vi "niRFUtil RFHS Channelizer FineTuneResamplerArray CSG.vi"(0 "Resampler Ref":refnum<data-value>, 1 "Data":csg[](array[numeric]), 2 "Data Subset":T1={"Offset"=0, "Length"=-1}, 4 "fs shift (ppm)":dbl, 5 "error in (no error)":errorcluster, 6 "Reset":bool, 7 "phase shift (samples)":dbl, 8 "Requested Output Samples":i32=-1, 10 "Benchmark Task":T2, 11 "CPU Context":string) -> (14 "Resampler Ref (out)":refnum<data-value>, 15 "Resampled Data":csg[](array[numeric]), 16 "Input Samples Consumed":i32, 19 "error out":errorcluster)   [LabVIEW 2015, in "niRFUtil.lvlib"]
uses:
  niRFUtil.lvlib
  Utilities/Benchmark/niRFUtil RFHS Benchmark Task.ctl
  Utilities/niRFUtil RFHS Util Data Subset.ctl
  Includes/niRFUtil RFHS Channelizer ResamplerInfo CSG.ctl
  Includes/niRFUtil RFHS Channelizer FilterRef.ctl
  Includes/niRFUtil RFHS Channelizer ChannelizerBufferingMode.ctl
  Utilities/Data FIFO/niRFUtil RFHS FIFO Reference.ctl
  Utilities/Data FIFO/niRFUtil RFHS FIFO.ctl
  Includes/niRFUtil RFHS Channelizer ChannelizerFlags.ctl
  niRFUtil RFHS Channelizer AdjustDataSubsetSpecification.vi
  Utilities/niRFUtil RFHS Util Dll Path.vi
  niRFUtil RFHS Channelizer ProcessCPUContext.vi
  niRFUtil RFHS Channelizer ChannelizerHandleDllError.vi
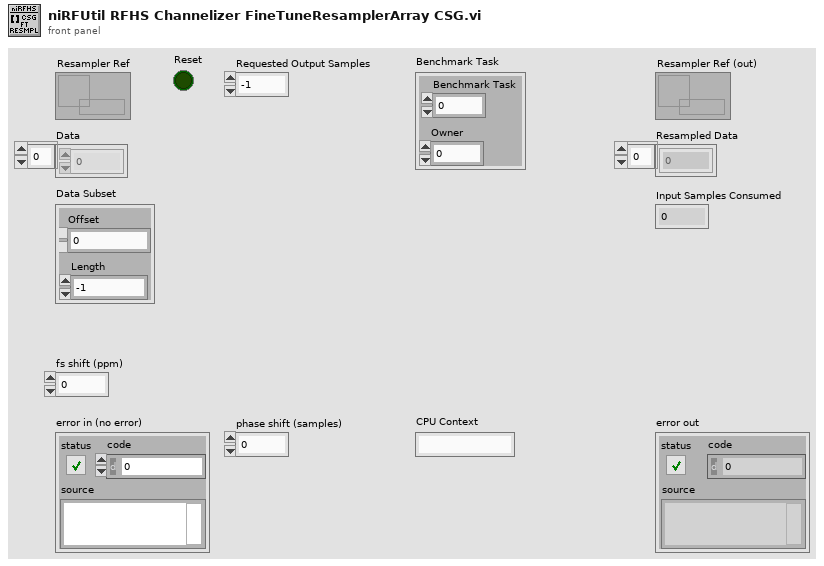
[diagram p1: front panel]
types:
  T1 = typedef "niRFUtil.lvlib/niRFUtil RFHS Util Data Subset.ctl" = cluster{"Offset":i32, "Length":i32}
  T2 = typedef "niRFUtil.lvlib/niRFUtil RFHS Benchmark Task.ctl" = cluster{"Benchmark Task":u64, "Owner":u32}
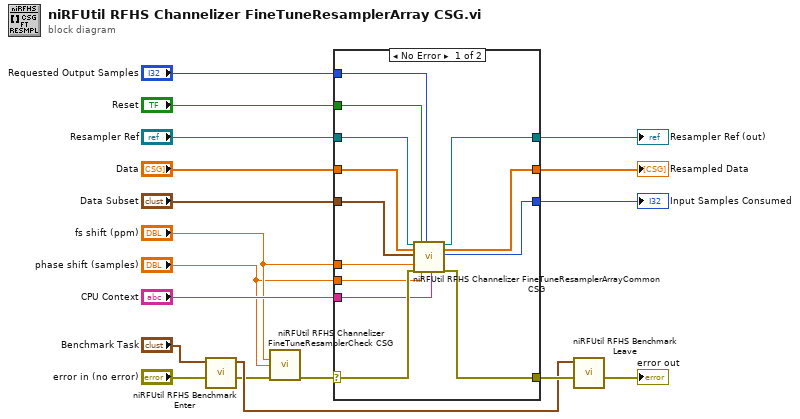
[diagram p0: block diagram]
diagram:
  n1 = call "niRFUtil RFHS Benchmark Enter.vi"("error in (no error)"="error in (no error)", "Benchmark Task (Parent)"="Benchmark Task") -> ("error out"=w4:errorcluster, "Benchmark Task (Self)"=w9:T2)  [unwired: 8 in]
  n2 = call "niRFUtil RFHS Channelizer FineTuneResamplerCheck CSG.vi"("fs shift (ppm)"="fs shift (ppm)", "phase shift (samples)"="phase shift (samples)", "error in (no error)"=w4) -> ("error out"=w3:errorcluster)  [unwired: 12 in]
  n3 = case shown="No Error" w3 {
    selector: w3 -> [w31 w33]
    tunnel: "Data" -> [w26 _]
    tunnel: "Reset" -> [w24 _]
    tunnel: [w21 w33] -> w15
    tunnel: [w22 _] -> w12
    tunnel: "CPU Context" -> [w30 _]
    tunnel: "Data Subset" -> [w27 _]
    tunnel: "Resampler Ref" -> [w29 w32]
    tunnel: [w28 w32] -> w7
    tunnel: "phase shift (samples)" -> [w23 _]
    tunnel: "fs shift (ppm)" -> [w25 _]
    tunnel: "Requested Output Samples" -> [w19 _]
    tunnel: [w20 _] -> w5
    frame No Error {
      n4 = call "niRFUtil RFHS Channelizer FineTuneResamplerArrayCommon CSG.vi"("Resampler Ref"=w29, "Data"=w26, "Data Subset"=w27, "fs shift (ppm)"=w25, "error in (no error)"=w31, "Reset"=w24, "phase shift (samples)"=w23, "Requested Output Samples"=w19, "CPU Context"=w30) -> ("Resampler Ref (out)"=w28:refnum<data-value>, "Resampled Data"=w22:csg[], "Input Samples Consumed"=w20:i32, "error out"=w21:errorcluster)  [unwired: 6 in, 1 out]
    }
    frame Error {
    }
  }
  "Resampled Data" <- w12
  "Resampler Ref (out)" <- w7
  "Input Samples Consumed" <- w5
  n5 = call "niRFUtil RFHS Benchmark Leave.vi"("error in (no error)"=w15, "Benchmark Task Self"=w9) -> ("error out"=→"error out":errorcluster)  [unwired: 8 in, 1 out]
